vi "to string.vi"(8 "error in":errorcluster, 11 "configuration in":refnum<class "RIO Target Configuration.lvclass">) -> (0 "error out":errorcluster, 1 "data":string, 2 "version":string, 3 "configuration out":refnum<class "RIO Target Configuration.lvclass">)   [LabVIEW 2014, in "RIO Target Configuration.lvclass"]
doc: "Provides an interface for saving a module configuration to a file or other serialized data source. It is recommended that all children of this class store data in two sets--data required for its own initialization, and any data required for parent initialization--and that each implementation uses the <b>Call Parent Method</b> primitive to serialize parent information."
uses:
  RIO Target Configuration.lvclass
  RIO Target Configuration.lvclass/RIO Target Configuration.ctl
  <vilib>/NI/Configuration Framework/serializable configuration/NISE_CEF_serializable configuration.lvclass
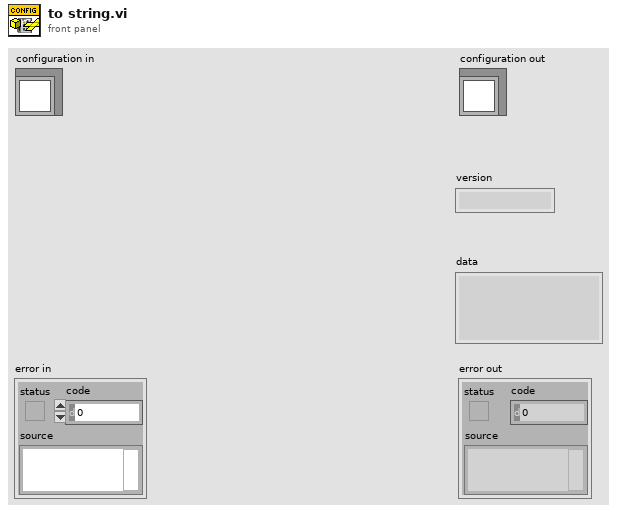
[diagram p1: front panel]
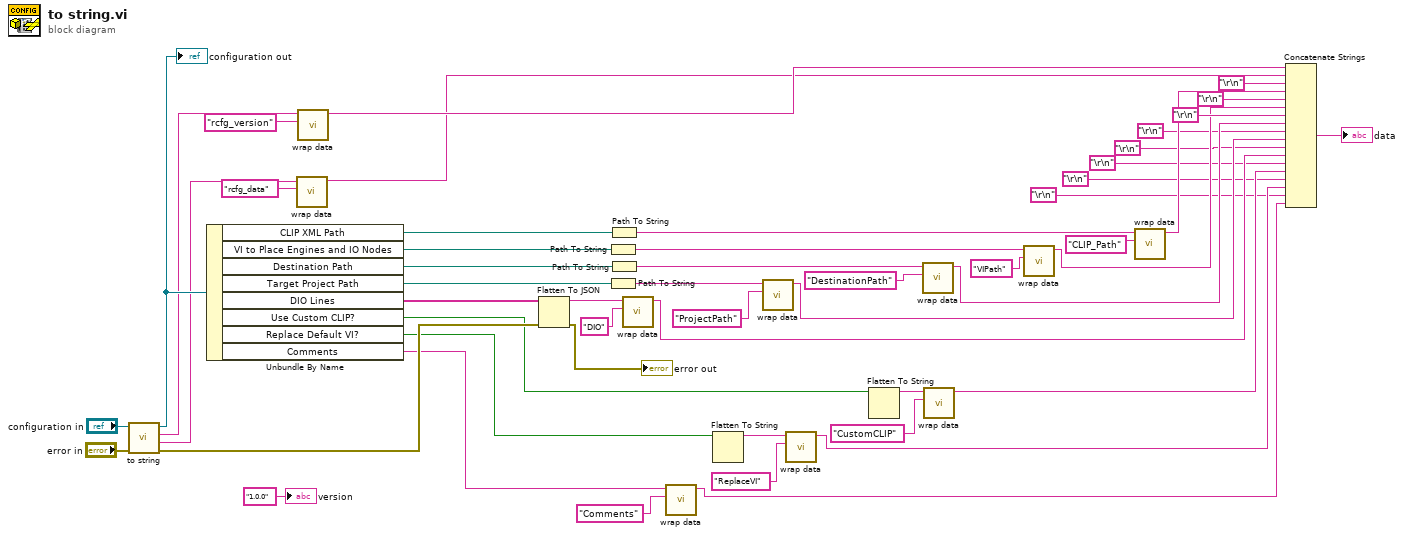
[diagram p0: block diagram]
diagram:
  n1 = call-parent "to string.vi"("error in"="error in", "configuration in"="configuration in") -> ("error out"=w44:errorcluster, "data"=w31:string, "version"=w30:string, "configuration out"=w47:refnum<class "RIO Target Configuration.lvclass">)  [unwired: 6 in]
  "configuration out" <- w47
  n2 = Unbundle By Name(w47) -> ("CLIP XML Path"=w33:path, "VI to Place Engines and IO Nodes"=w36:path, "Destination Path"=w39:path, "Target Project Path"=w42:path, "DIO Lines"=w45:string[], "Use Custom CLIP?"=w14:bool, "Replace Default VI?"=w12:bool, "Comments"=w10:string)
  n3 = call <vilib>:"wrap data.vi"("identifier"="rcfg_data", "data to wrap"=w31) -> ("wrapped data"=w24:string)  [unwired: 9 in]
  n4 = call <vilib>:"wrap data.vi"("identifier"="rcfg_version", "data to wrap"=w30) -> ("wrapped data"=w25:string)  [unwired: 9 in]
  n5 = Flatten To JSON(anything=w45, error in (no error)=w44) -> (JSON string=w43:string, 11:→"error out":errorcluster)  [unwired: 1 in]
  n6 = Path To String(path=w36) -> (string=w35:string)
  n7 = Path To String(path=w42) -> (string=w41:string)
  n8 = Path To String(path=w33) -> (string=w32:string)
  n9 = Path To String(path=w39) -> (string=w37:string)
  n10 = call <vilib>:"wrap data.vi"("identifier"="DIO" ("key"), "data to wrap"=w43) -> ("wrapped data"=w17:string)  [unwired: 9 in]
  n11 = call <vilib>:"wrap data.vi"("identifier"="Comments", "data to wrap"=w10) -> ("wrapped data"=w1:string)  [unwired: 9 in]
  n12 = Flatten To String(anything=w12) -> (data string=w11:string)  [unwired: 3 in, 2 out]
  n13 = call <vilib>:"wrap data.vi"("identifier"="ProjectPath" ("key"), "data to wrap"=w41) -> ("wrapped data"=w19:string)  [unwired: 9 in]
  n14 = call <vilib>:"wrap data.vi"("identifier"="ReplaceVI", "data to wrap"=w11) -> ("wrapped data"=w3:string)  [unwired: 9 in]
  n15 = Flatten To String(anything=w14) -> (data string=w13:string)  [unwired: 3 in, 2 out]
  n16 = call <vilib>:"wrap data.vi"("identifier"="DestinationPath" ("key"), "data to wrap"=w37) -> ("wrapped data"=w21:string)  [unwired: 9 in]
  n17 = call <vilib>:"wrap data.vi"("identifier"="CustomCLIP", "data to wrap"=w13) -> ("wrapped data"=w5:string)  [unwired: 9 in]
  n18 = call <vilib>:"wrap data.vi"("identifier"="VIPath" ("key"), "data to wrap"=w35) -> ("wrapped data"=w22:string)  [unwired: 9 in]
  n19 = call <vilib>:"wrap data.vi"("identifier"="CLIP_Path" ("key"), "data to wrap"=w32) -> ("wrapped data"=w23:string)  [unwired: 9 in]
  n20 = Concatenate Strings(w25, w24, "\r\n", w23, "\r\n", w22, "\r\n", w21, "\r\n", w19, "\r\n", w17, "\r\n", w5, "\r\n", w3, "\r\n", w1) -> (→"data":string)
  "version" <- "1.0.0" ("version")
